vi "Gamma_s_2024.vi"(2 "CO2 content (ppm)":dbl=542.0, 3 "xw molar fraction of water vapor":dbl=0.013091, 4 "Type of air":i32(listbox)=4) -> (0 "Gamma_s Zuckerwar (wrong)":dbl=1.3989554548281689 format="%_6g", 1 "Gamma_s correct":dbl=1.40043330947759 format="%.6g")   [LabVIEW 2016]
uses:
  2022/SOS_Global_2022.vi
panel:
  out "rel. diff. CP0 diatomic / ppm":dbl=-2678.131911934556
  out "CP0/R dry":dbl=3.490626538308229
  out "rel. diff. gamma0 correct - Zuck (ppm)":dbl=1056.398646805068
  out "xCH4":dbl=1.999543856771026e-06 format="%_3g"
  out "xKr":dbl=1.139739998359485e-06 format="%_3g"
  out "xHe":dbl=5.238804904740088e-06 format="%_3g"
  out "xNe":dbl=1.8175853658048626e-05 format="%_3g"
  out "xCO2":dbl=0.000542 format="%_6g"
  out "xAr":dbl=0.009337869811120692 format="%.7g"
  out "xO2":dbl=0.20942822447048373 format="%_7g"
  out "xN2":dbl=0.780661912560544 format="%_7g"
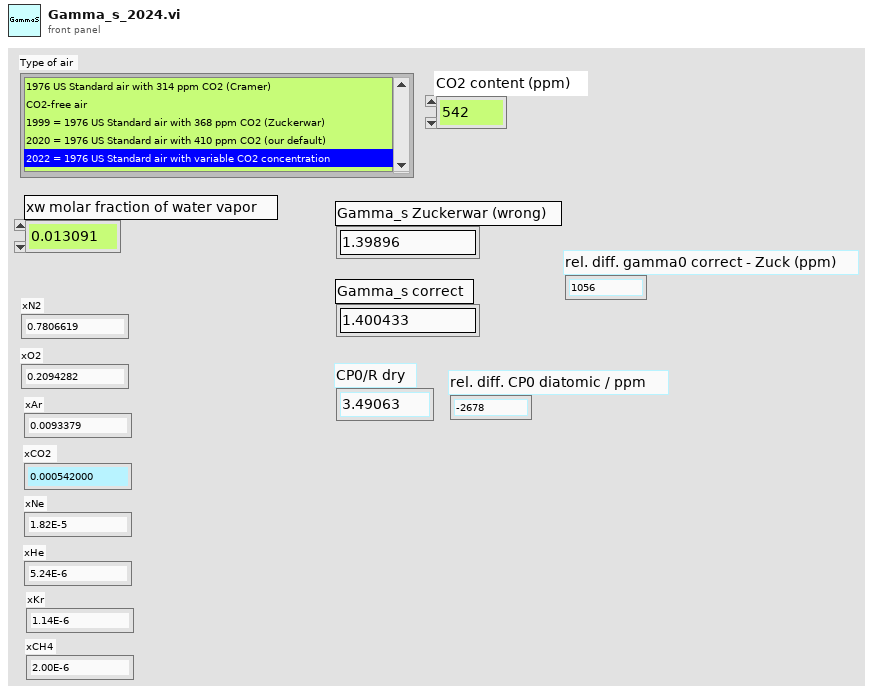
[diagram p1: front panel]
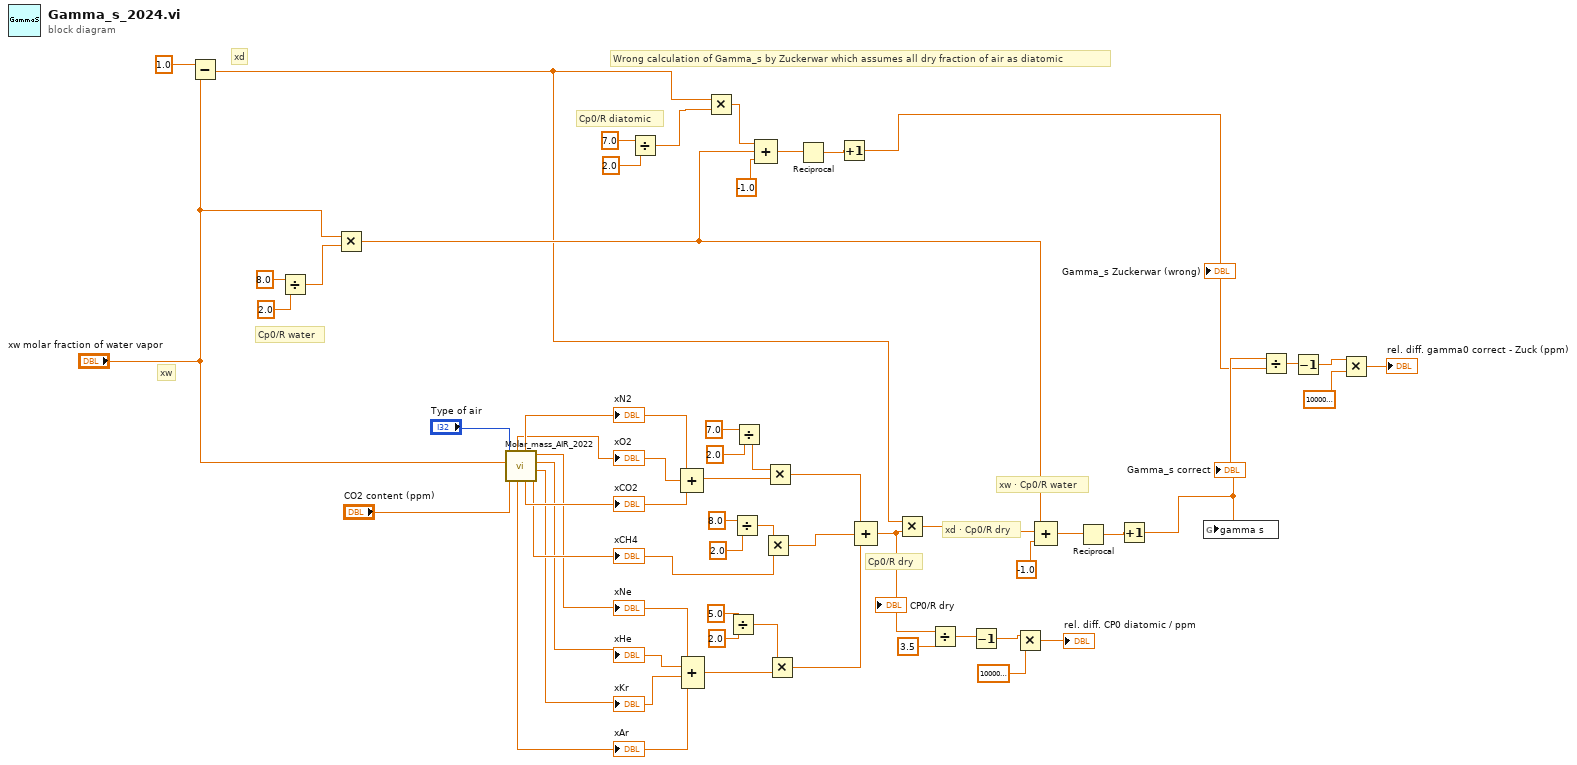
[diagram p0: block diagram]
diagram:
  # "Wrong calculation of Gamma_s by Zuckerwar which assumes all dry fraction of air as diatomic"
  # "xd · Cp0/R dry"
  # "xw · Cp0/R water"
  # "Cp0/R dry"
  # "xd"
  # "xw"
  # "Cp0/R water"
  # "Cp0/R diatomic"
  n1 = Subtract(x=1.0, y="xw molar fraction of water vapor") -> (x-y=w14:dbl)
  n2 = Divide(x=8.0, y=2.0) -> (x/y=w47:dbl)
  n3 = Multiply(x="xw molar fraction of water vapor", y=w47) -> (x*y=w15:dbl)
  n4 = call "Molar_mass_AIR_2022.vi"("CO2 content (ppm)"="CO2 content (ppm)", "xw molar fraction of water vapor"="xw molar fraction of water vapor", "Type of air"="Type of air") -> ("xCH4"=w32:dbl, "xKr"=w28:dbl, "xHe"=w29:dbl, "xNe"=w30:dbl, "xCO2"=w36:dbl, "xN2"=w38:dbl, "xAr"=w27:dbl, "xO2"=w37:dbl)  [unwired: 1 out]
  "xN2" <- w38
  "xO2" <- w37
  "xAr" <- w27
  "xCO2" <- w36
  "xNe" <- w30
  "xHe" <- w29
  "xKr" <- w28
  "xCH4" <- w32
  n5 = Divide(x=7.0, y=2.0) -> (x/y=w51:dbl)
  n6 = Compound Arithmetic op=ADD(w38, w37, w36) -> (w35:dbl)
  n7 = Compound Arithmetic op=ADD(w30, w29, w28, w27) -> (w23:dbl)
  n8 = Multiply(x=w14, y=w51) -> (x*y=w50:dbl)
  n9 = Divide(x=5.0, y=2.0) -> (x/y=w24:dbl)
  n10 = Divide(x=8.0, y=2.0) -> (x/y=w31:dbl)
  n11 = Divide(x=7.0, y=2.0) -> (x/y=w39:dbl)
  n12 = Compound Arithmetic op=ADD(w50, w15, -1.0 ("value")) -> (w45:dbl)
  n13 = Multiply(x=w31, y=w32) -> (x*y=w21:dbl)
  n14 = Multiply(x=w39, y=w35) -> (x*y=w22:dbl)
  n15 = Multiply(x=w24, y=w23) -> (x*y=w20:dbl)
  n16 = Reciprocal(x=w45) -> (1/x=w19:dbl)
  n17 = Increment(x=w19) -> (x+1=w11:dbl)
  "Gamma_s Zuckerwar (wrong)" <- w11
  n18 = Compound Arithmetic op=ADD(w22, w21, w20) -> (w6:dbl)
  "CP0/R dry" <- w6
  n19 = Multiply(x=w14, y=w6) -> (x*y=w13:dbl)
  n20 = Divide(x=w6, y=3.5) -> (x/y=w4:dbl)
  n21 = Decrement(x=w4) -> (x-1=w3:dbl)
  n22 = Multiply(x=w3, y=1000000.0) -> (x*y=→"rel. diff. CP0 diatomic / ppm":dbl)
  n23 = Compound Arithmetic op=ADD(w15, w13, -1.0 ("value")) -> (w17:dbl)
  n24 = Reciprocal(x=w17) -> (1/x=w16:dbl)
  n25 = Increment(x=w16) -> (x+1=w12:dbl)
  "Gamma_s correct" <- w12
  n26 = global write "SOS_Global_2022.vi" "gamma s"(w12) -> ()
  n27 = Divide(x=w12, y=w11) -> (x/y=w10:dbl)
  n28 = Decrement(x=w10) -> (x-1=w9:dbl)
  n29 = Multiply(x=w9, y=1000000.0) -> (x*y=→"rel. diff. gamma0 correct - Zuck (ppm)":dbl)
